vi "Acceleration from Velocities and Time.vi"(9 "Time (s)":dbl, 10 "Final Velocity (in/s)":dbl, 11 "Initial Velocity (in/s)":dbl) -> (3 "Acceleration (in/s2)":dbl)   [LabVIEW 2019, in "Motion Profile Generator.lvclass"]
uses:
  Motion Profile Generator.lvclass
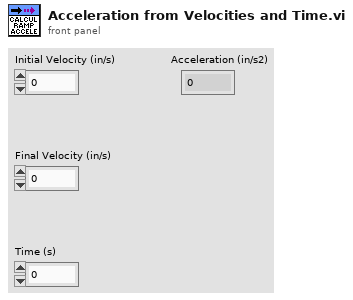
[diagram p1: front panel]
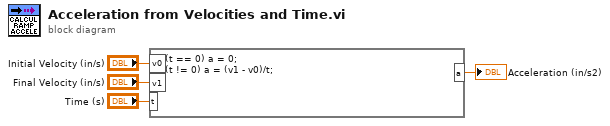
[diagram p0: block diagram]
diagram:
  n1 = formula code="if(t == 0) a = 0;\nif(t != 0) a = (v1 - v0)/t;"("v0"="Initial Velocity (in/s)", "v1"="Final Velocity (in/s)", "t"="Time (s)") -> ("a"=→"Acceleration (in/s2)":dbl)
